vi "control loop update execution timing tag.vi"(7 "tag to update":T2, 8 "use external value? (F)":bool, 9 "value (0)":dbl, 10 "execution inidces in":T1, 11 "control loop data in":T4) -> (2 "execution inidces out":T1, 3 "control loop data out":T4)   [LabVIEW 2013, in "main engine.lvlib"]
doc: "This VI can be used to write any engine-relate metrics required before the current cycle's module execution begins."
uses:
  main engine.lvlib
  control loop data.ctl
  <vilib>/NI/Tag Bus/table/data table.ctl
  engine run schedule.ctl
  engine decimation schedule.ctl
  full module data.ctl
  <vilib>/NI/Tag Bus Module Framework/runtime/TBM module execution interface.lvclass
  module run state.ctl
  async executor/asynchronous executor reference.ctl
  async executor/async message to executor.ctl
  Runtime/async command notification.ctl
  Runtime/async error info.ctl
  <vilib>/NI/Tag Bus Module Framework/runtime/error classification.ctl
  <vilib>/NI/Tag Bus Module Framework/module configuration/TBM module configuration.lvclass
  module method data.ctl
  <vilib>/NI/Tag Bus/table/transfer specification.ctl
  <vilib>/NI/Tag Bus/tag/Data Type.ctl
  fault handling spec.ctl
  Configuration/Error Actions.ctl
  execution timing indices.ctl
  pre-execution data.ctl
  execution time fields.ctl
  <vilib>/NI/Tag Bus/table/data polymorphs/write one/write Double.vi
  <vilib>/NI/Tag Bus/table/data table.lvlib
  <vilib>/NI/Tag Bus/tag/tag descriptor.lvclass
  Configuration/Standard Engine Configuration.lvclass
panel:
  out "execution timing out":T3
  in  "execution timing in":T3
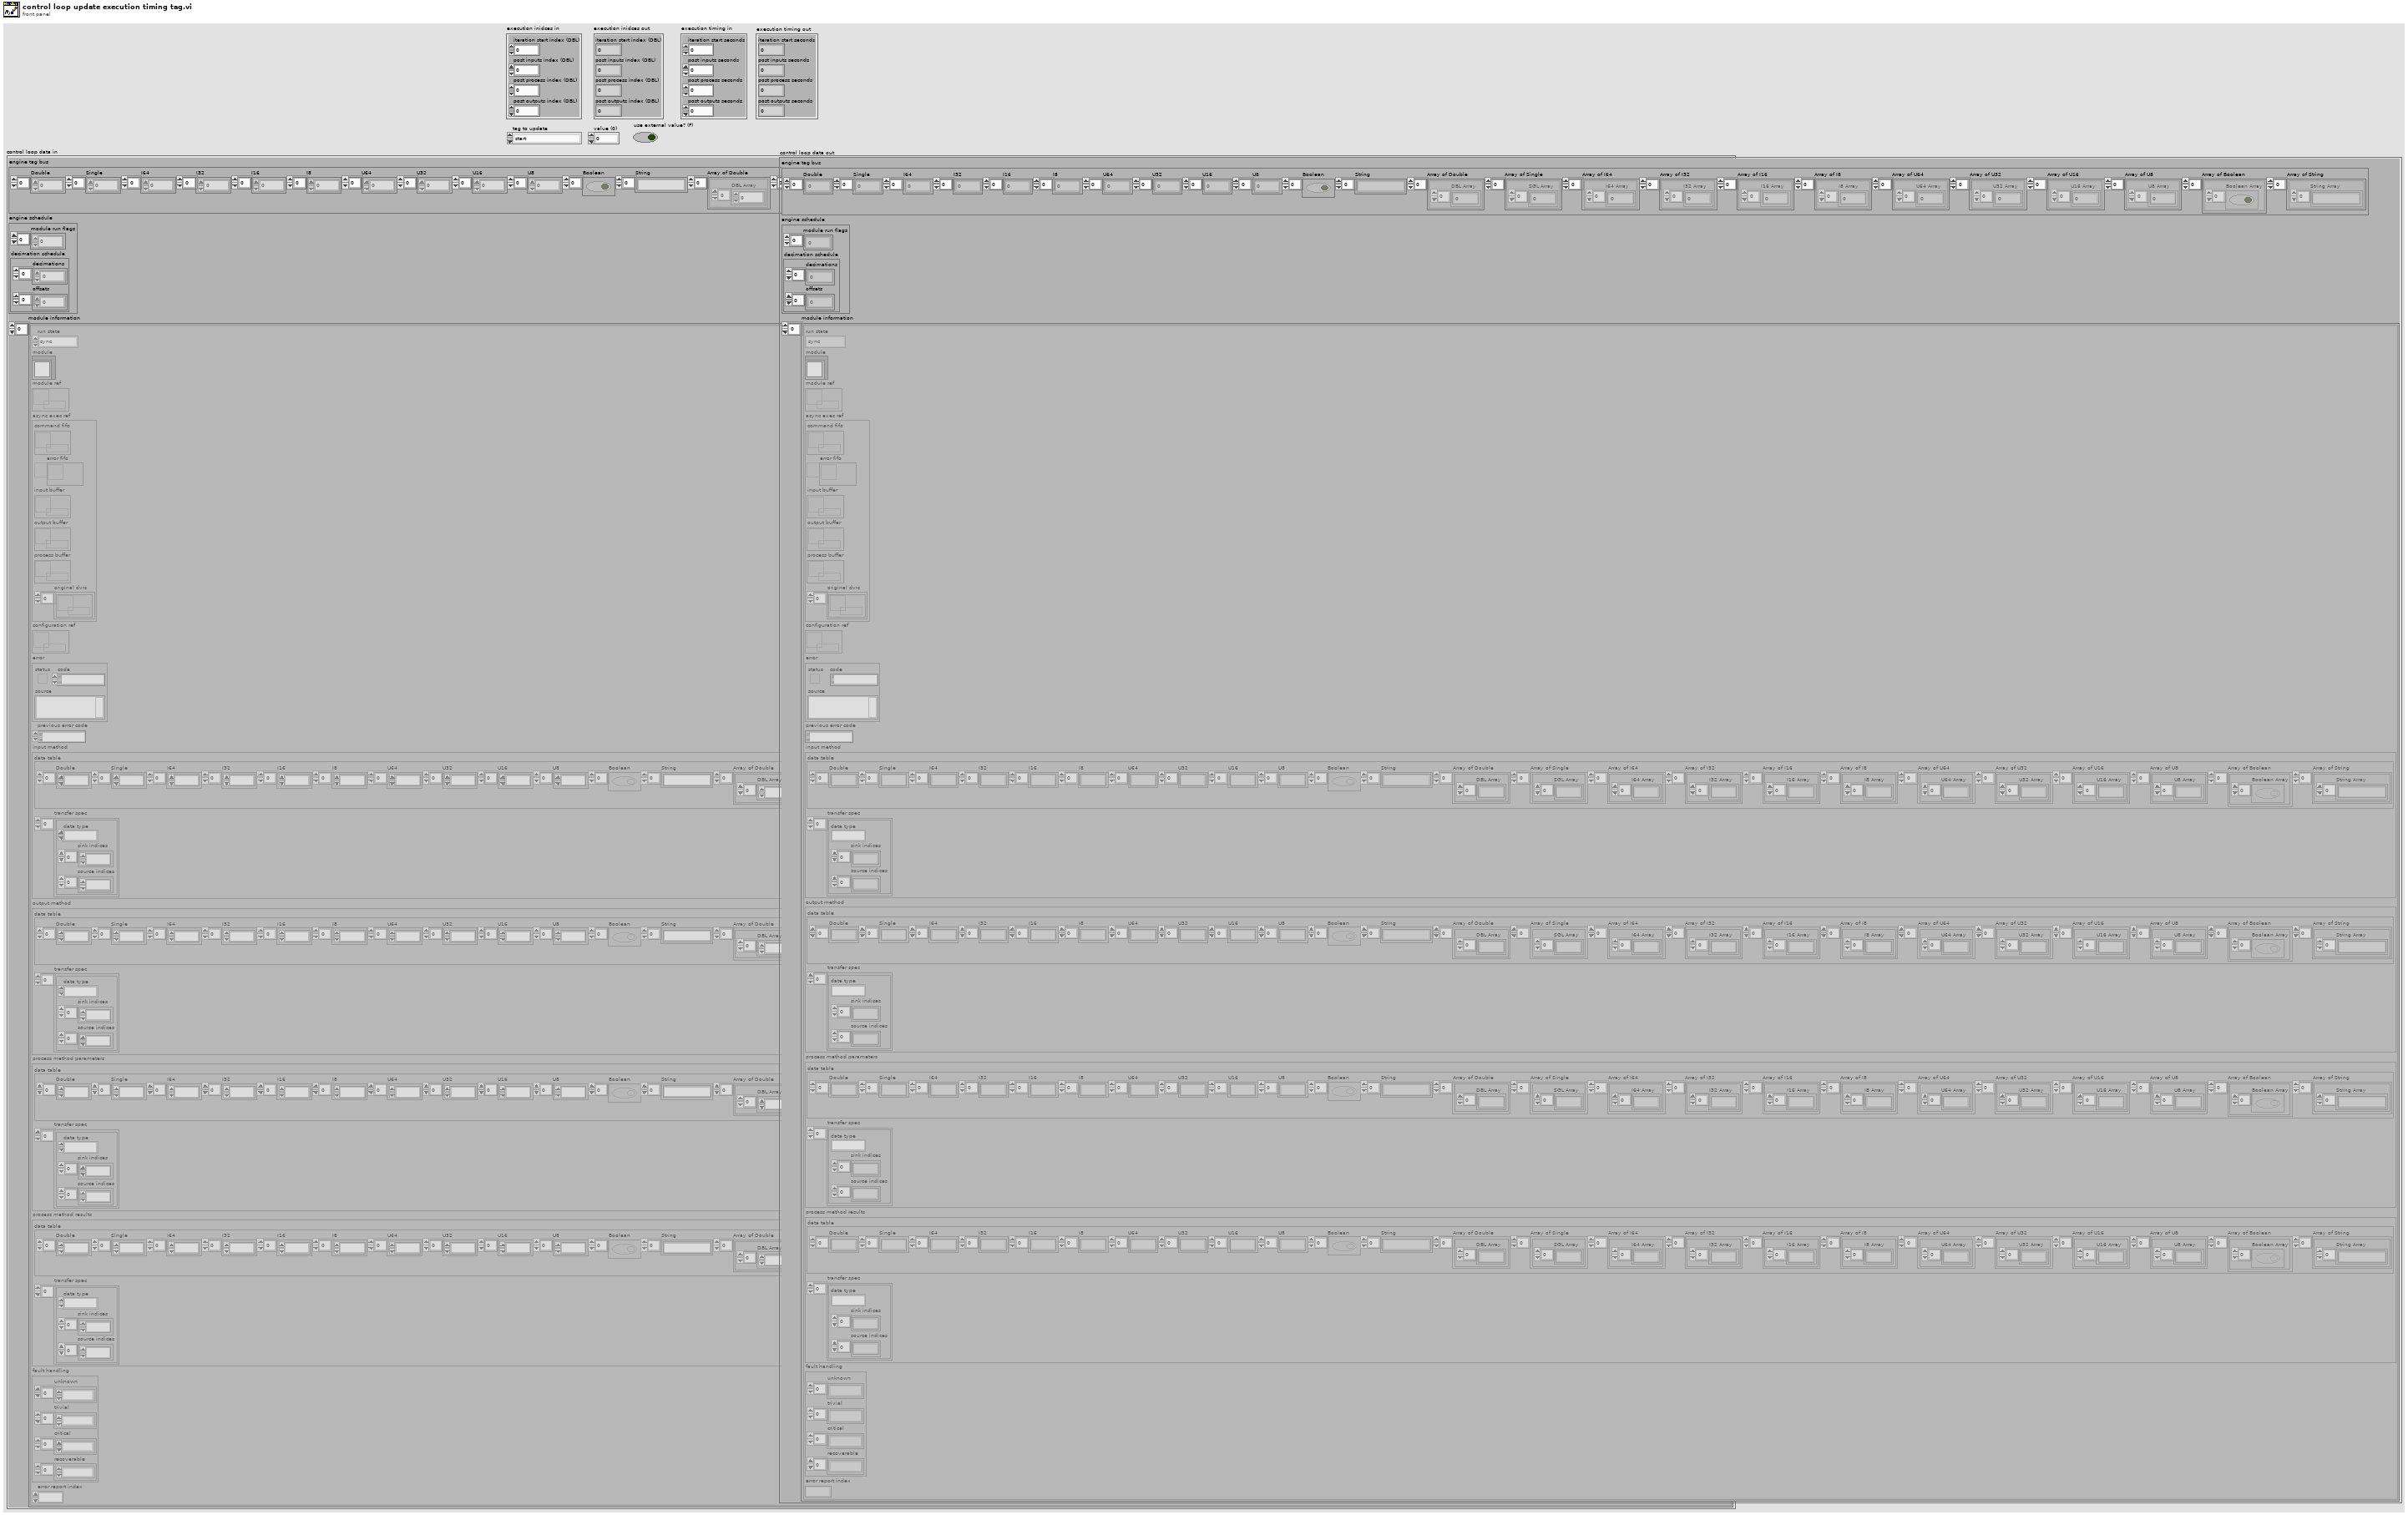
[diagram p1: front panel]
types:
  T1 = typedef "main engine.lvlib/execution timing indices.ctl" = cluster{"iteration start index (DBL)":i32, "post inputs index (DBL)":i32, "post process index (DBL)":i32, "post outputs index (DBL)":i32}
  T2 = typedef "main engine.lvlib/execution time fields.ctl" = enum16{"start", "inputs", "process", "outputs"}
  T3 = typedef "main engine.lvlib/pre-execution data.ctl" = cluster{"iteration start seconds":dbl, "post inputs seconds":dbl, "post process seconds":dbl, "post outputs seconds":dbl}
  T4 = typedef "main engine.lvlib/control loop data.ctl" = cluster{"engine tag bus":T5, "engine schedule":T6, "module information":T8[]}
  T5 = typedef "tag bus.lvlib/data table.lvlib/data table.ctl" = cluster{"Double":dbl[], "Single":sgl[], "I64":i64[], "I32":i32[], "I16":i16[], "I8":i8[], "U64":u64[], "U32":u32[], "U16":u16[], "U8":u8[], "Boolean":bool[], "String":string[], "Array of Double":cluster{"DBL Array":dbl[]}[], "Array of Single":cluster{"SGL Array":sgl[]}[], "Array of I64":cluster{"I64 Array":i64[]}[], "Array of I32":cluster{"I32 Array":i32[]}[], "Array of I16":cluster{"I16 Array":i16[]}[], "Array of I8":cluster{"I8 Array":i8[]}[], "Array of U64":cluster{"U64 Array":u64[]}[], "Array of U32":cluster{"U32 Array":u32[]}[], "Array of U16":cluster{"U16 Array":u16[]}[], "Array of U8":cluster{"U8 Array":u8[]}[], "Array of Boolean":cluster{"Boolean Array":bool[]}[], "Array of String":cluster{"String Array":string[]}[]}
  T6 = typedef "main engine.lvlib/engine run schedule.ctl" = cluster{"module run flags":u8[], "decimation schedule":T7}
  T7 = typedef "main engine.lvlib/engine decimation schedule.ctl" = cluster{"decimations":u16[], "offsets":u16[]}
  T8 = typedef "main engine.lvlib/full module data.ctl" = cluster{"run state":T9, "module":refnum<class "TBM module execution interface.lvclass">, "module ref":refnum<data-value>, "async exec ref":T10, "configuration ref":refnum<data-value>, "error":errorcluster, "previous error code":i32, "input method":T11, "output method":T11, "process method parameters":T11, "process method results":T11, "fault handling":T14, "error report index ":i32}
  T9 = typedef "main engine.lvlib/module run state.ctl" = enum16{"sync", "async"}
  T10 = typedef "main engine.lvlib/asynchronous executor reference.ctl" = cluster{"command fifo":refnum<k33>, "error fifo":refnum<k33>, "input buffer":refnum<k33>, "output buffer":refnum<k33>, "process buffer":refnum<k33>, "original dvrs":refnum<data-value>[]}
  T11 = typedef "main engine.lvlib/module method data.ctl" = cluster{"data table":T5, "transfer spec":T12[]}
  T12 = typedef "tag bus.lvlib/data table.lvlib/transfer specification.ctl" = cluster{"data type":T13, "sink indices":i32[], "source indices":i32[]}
  T13 = typedef "tag bus.lvlib/tag descriptor.lvclass/Data Type.ctl" = enum16{"Double", "Single", "I64", "I32", "I16", "I8", "U64", "U32", "U16", "U8", "Boolean", "String", "Array of Double", "Array of Single", "Array of I64", "Array of I32", "Array of I16", "Array of I8", "Array of U64", "Array of U32", "Array of U16", "Array of U8", "Array of Boolean", "Array of String"}
  T14 = typedef "main engine.lvlib/fault handling spec.ctl" = cluster{"unknown":T15[], "trivial":T15[], "critical":T15[], "recoverable":T15[]}
  T15 = typedef "Standard Engine Configuration.lvclass/Error Actions.ctl" = enum16{"Clear", "Notify", "Log", "Stop Component", "Stop Engine", "Safe State", "Attempt Recovery"}
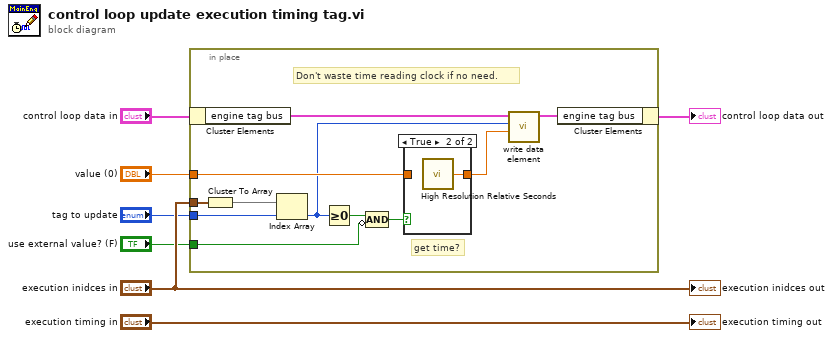
[diagram p0: block diagram]
diagram:
  n1 = in-place {
    in-place-border: "execution inidces in" -> [w16]
    in-place-border: "tag to update" -> [w14]
    in-place-border: "value (0)" -> [w13]
    in-place-border: "use external value? (F)" -> [w9]
    # "Don't waste time reading clock if no need."
    # "get time?"
    n2 = in-place-cluster #1("control loop data in") -> ("engine tag bus"=w18:T5)
    n3 = Cluster To Array(cluster=w16) -> (array=w15:i32[])
    n4 = Index Array(array=w15, index=w14) -> (element=w10:i32)
    n5 = Greater Or Equal To 0?(x=w10) -> (x >= 0?=w12:bool)
    n6 = Compound Arithmetic op=AND(w12, invert w9) -> (w11:bool)
    n7 = case shown="True" w11 {
      tunnel: [w19 w20] -> w8
      tunnel: w13 -> [w19 _]
      frame False {
      }
      frame True {
        n8 = call <vilib>:"High Resolution Relative Seconds.vi"() -> ("relative seconds"=w20:dbl)
      }
    }
    n9 = call-poly <vilib>:"write data element.vi"("value"=w8, "index"=w10, "data table in"=w18) -> ("data table out"=w17:T5)  [unwired: 8 in]
    n10 = in-place-cluster #1("engine tag bus"=w17) -> (→"control loop data out":T4)
  }
  "execution timing out" <- "execution timing in"
  "execution inidces out" <- "execution inidces in"
